vi "Generate R(theta).vi"(1 "Axis":enum16{"x", "y", "z"}(ring), 3 "Angle (degrees)":dbl=45.0 format="%.2f") -> (0 "Screw":T2=[[1.0, 0.0, 0.0, 0.0], [0.0, 1.0, 0.0, 0.0], [0.0, 0.0, 1.0, 0.0], [0.0, 0.0, 0.0, 1.0]])   [LabVIEW 2018]
uses:
  <vilib>/Analysis/Matrix/Datatypes/RealMatrix.ctl
  <vilib>/Analysis/Matrix/NI_Matrix.lvlib
panel:
  in  "Default":T1={"nx"=1.0, "ny"=0.0, "nz"=0.0, "nw"=0.0, "ox"=0.0, "oy"=1.0, "oz"=0.0, "ow"=0.0, "ax"=0.0, "ay"=0.0, "az"=1.0, "aw"=0.0, "Px"=0.0, "Py"=0.0, "Pz"=0.0, "Pw"=1.0} {"Pw" format="%.2f"; "Pz" format="%.2f"; "Py" format="%.2f"; "Px" format="%.2f"; "aw" format="%.2f"; "az" format="%.2f"; "ay" format="%.2f"; "ax" format="%.2f"; "ow" format="%.2f"; "nw" format="%.2f"; "oz" format="%.2f"; "oy" format="%.2f"; "ox" format="%.2f"; "nz" format="%.2f"; "ny" format="%.2f"; "nx" format="%.2f"}
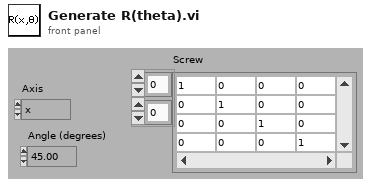
[diagram p1: front panel]
types:
  T1 = cluster{"nx":dbl, "ny":dbl, "nz":dbl, "nw":dbl, "ox":dbl, "oy":dbl, "oz":dbl, "ow":dbl, "ax":dbl, "ay":dbl, "az":dbl, "aw":dbl, "Px":dbl, "Py":dbl, "Pz":dbl, "Pw":dbl}
  T2 = typedef "NI_Matrix.lvlib/RealMatrix.ctl" = dbl[][]
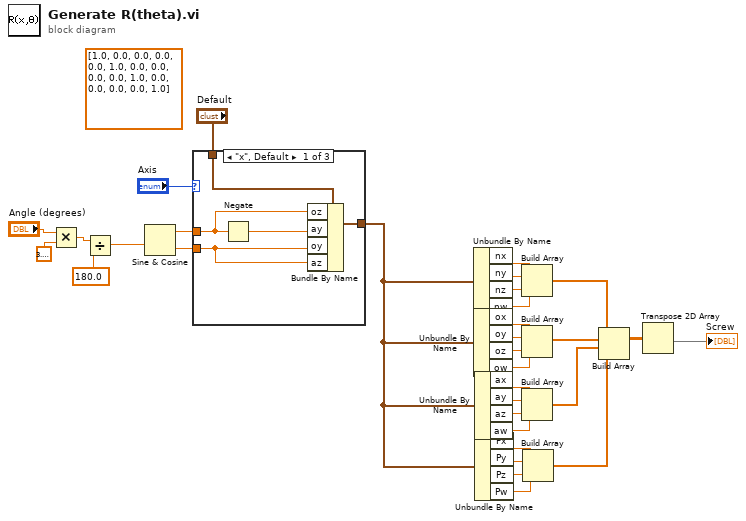
[diagram p0: block diagram]
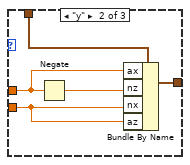
[diagram p2: hidden frame]
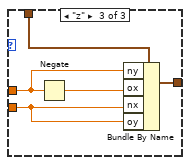
[diagram p3: hidden frame]
diagram:
  (unwired) T2 [[1.0, 0.0, 0.0, 0.0], [0.0, 1.0, 0.0, 0.0], [0.0, 0.0, 1.0, 0.0], [0.0, 0.0, 0.0, 1.0]] ("Start")
  n1 = Multiply(x="Angle (degrees)", y=3.141592653589793) -> (x*y=w30:dbl)
  n2 = Divide(x=w30, y=180.0) -> (x/y=w26:dbl)
  n3 = Sine & Cosine(0:w26) -> (1:w24:dbl, 2:w25:dbl)
  n4 = case shown="\"x\", Default" "Axis" {
    tunnel: "Default" -> [w37 w42 w47]
    tunnel: [w36 w41 w46] -> w2
    tunnel: w25 -> [w33 w38 w43]
    tunnel: w24 -> [w34 w39 w44]
    frame "x", Default {
      n5 = Negate(x=w34) -> (-x=w35:dbl)
      n6 = Bundle By Name(cluster=w37, "oz"=w34, "ay"=w35, "oy"=w33, "az"=w33) -> (w36:T1)
    }
    frame "y" {
      n7 = Negate(x=w39) -> (-x=w40:dbl)
      n8 = Bundle By Name(cluster=w42, "ax"=w39, "nz"=w40, "nx"=w38, "az"=w38) -> (w41:T1)
    }
    frame "z" {
      n9 = Negate(x=w44) -> (-x=w45:dbl)
      n10 = Bundle By Name(cluster=w47, "ny"=w44, "ox"=w45, "nx"=w43, "oy"=w43) -> (w46:T1)
    }
  }
  n11 = Unbundle By Name(w2) -> ("nx"=w15:dbl, "ny"=w16:dbl, "nz"=w17:dbl, "nw"=w14:dbl)
  n12 = Unbundle By Name(w2) -> ("ox"=w20:dbl, "oy"=w19:dbl, "oz"=w18:dbl, "ow"=w12:dbl)
  n13 = Unbundle By Name(w2) -> ("ax"=w21:dbl, "ay"=w22:dbl, "az"=w23:dbl, "aw"=w13:dbl)
  n14 = Unbundle By Name(w2) -> ("Px"=w11:dbl, "Py"=w10:dbl, "Pz"=w9:dbl, "Pw"=w8:dbl)
  n15 = Build Array(w15, w16, w17, w14) -> (w7:dbl[])
  n16 = Build Array(w20, w19, w18, w12) -> (w6:dbl[])
  n17 = Build Array(w21, w22, w23, w13) -> (w5:dbl[])
  n18 = Build Array(w11, w10, w9, w8) -> (w4:dbl[])
  n19 = Build Array(w7, w6, w5, w4) -> (w3:dbl[][])
  n20 = Transpose 2D Array(2D array=w3) -> (transposed array=→"Screw":dbl[][])
